vi "emi_Is Path.vi"(7 "Path":path) -> (8 "Path?":bool)   [LabVIEW 2011]
doc: "Verify that input is a valid Path. Does not check if path exists.\n\nReentrant Subroutine for throughput"
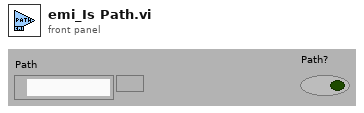
[diagram p1: front panel]
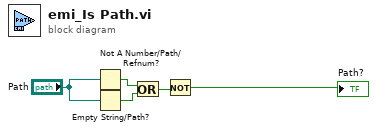
[diagram p0: block diagram]
diagram:
  n1 = Not A Number/Path/Refnum?(number/path/refnum="Path") -> (NaN/Path/Refnum?=w4:bool)
  n2 = Empty String/Path?(string/path="Path") -> (empty?=w3:bool)
  n3 = Or(x=w4, y=w3) -> (x .or. y?=w2:bool)
  n4 = Not(x=w2) -> (.not. x?=→"Path?":bool)
